vi "Read Paths.vi"(8 "error in (no error)":errorcluster, 11 "ParseXML in":refnum<class "ParseSVG.lvclass">) -> (0 "error out":errorcluster, 2 "Paths":T1[](array[typedef]), 3 "ParseXML out":refnum<class "ParseSVG.lvclass">)   [LabVIEW 2019, in "ParseSVG.lvclass"]
uses:
  ParseSVG.lvclass
  Path.ctl
  ParseSVG.lvclass/ParseSVG.ctl
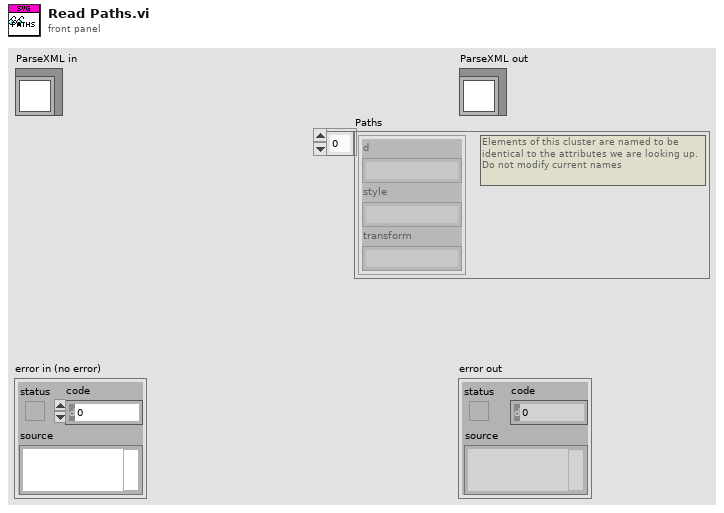
[diagram p1: front panel]
types:
  T1 = typedef "ParseSVG.lvclass/Path.ctl" = cluster{"d":string, "style":string, "transform":string}
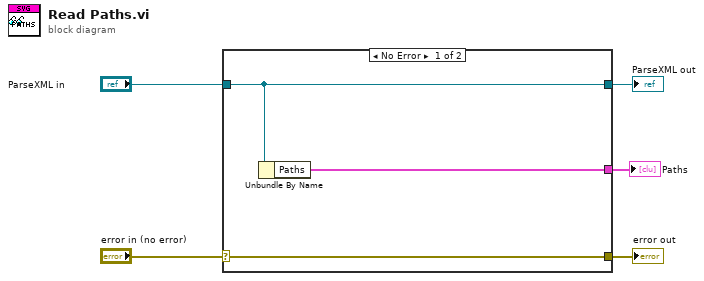
[diagram p0: block diagram]
diagram:
  n1 = case shown="No Error" "error in (no error)" {
    selector: "error in (no error)" -> [w8 w9]
    tunnel: [w8 w9] -> w4
    tunnel: [w7 w10] -> w2
    tunnel: "ParseXML in" -> [w7 w10]
    tunnel: [w6 _] -> w1
    frame No Error {
      n2 = Unbundle By Name(w7) -> ("Paths"=w6:T1[])
    }
    frame Error {
    }
  }
  "error out" <- w4
  "ParseXML out" <- w2
  "Paths" <- w1
